vi "Test Case, Charger_Wake-Up and Close.vi"(4 "error in":errorcluster) -> (0 "error out":errorcluster)   [LabVIEW 2010]
uses:
  Drivers/Charger Test Set/Charger_Input Control.ctl
panel:
  in  "Charger":T1={"address"="COM17", "position"=0, "setpoint"=7500.0} {"setpoint" min=0.0 max=20000.0 step=100.0; "position" min=0 max=5 step=1}
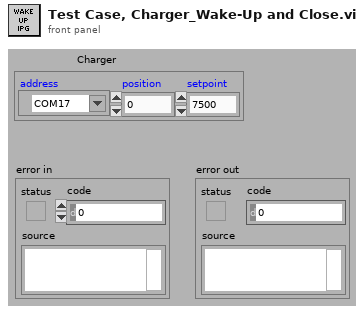
[diagram p1: front panel]
types:
  T1 = typedef "Charger_Input Control.ctl" = cluster{"address":refnum<visa-resource-name>, "position":i32, "setpoint":dbl}
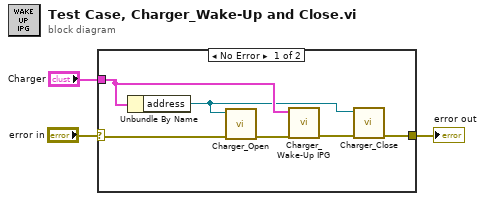
[diagram p0: block diagram]
diagram:
  n1 = case shown="No Error" "error in" {
    selector: "error in" -> [w6 w10]
    tunnel: [w7 w10] -> w3
    tunnel: "Charger" -> [w5 _]
    frame No Error {
      n2 = Unbundle By Name(w5) -> ("address"=w4:refnum<visa-resource-name>)
      n3 = call "Charger_Open.vi"("error in"=w6, "Charger COM port"=w4) -> ("error out"=w9:errorcluster)  [unwired: 5 in]
      n4 = call "Charger_Wake-Up IPG.vi"("error in"=w9, "Charger"=w5) -> ("error out"=w8:errorcluster)  [unwired: 7 in]
      n5 = call "Charger_Close.vi"("error in"=w8, "address"=w4) -> ("error out"=w7:errorcluster)  [unwired: 5 in]
    }
    frame Error {
    }
  }
  "error out" <- w3
